vi "GEOM_VAR_HeadersArray.vi"(9 "Action":T2, 10 "GEOM_HeadersArray":T1[](array[typedef])) -> (2 "GEOM_HeadersArray out":T1[](array[typedef]))   [LabVIEW 2016]
uses:
  GEOM_VAR_action.ctl
  GEOM_ReadModeHeader.ctl
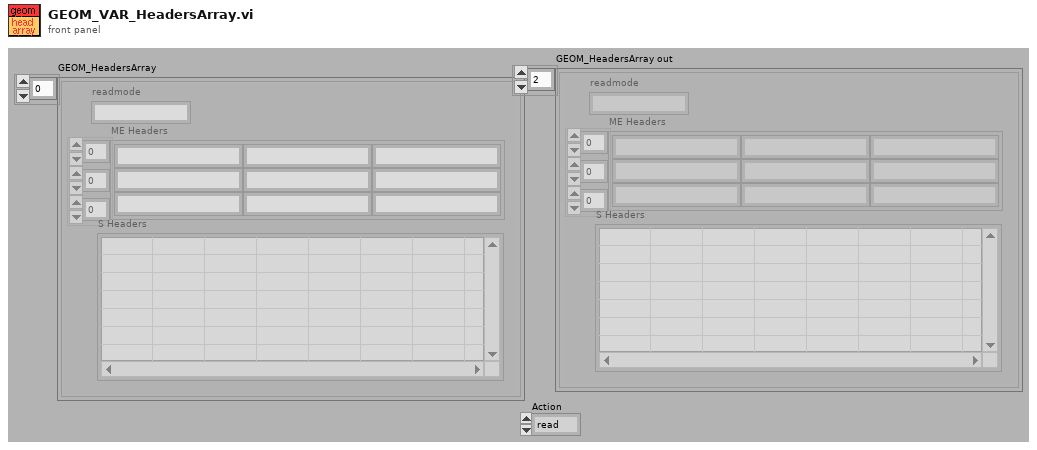
[diagram p1: front panel]
types:
  T1 = typedef "GEOM_ReadModeHeader.ctl" = cluster{"readmode":string, "ME Headers":string[][][], "S Headers":string[][]}
  T2 = typedef "GEOM_VAR_action.ctl" = enum16{"read", "write"}
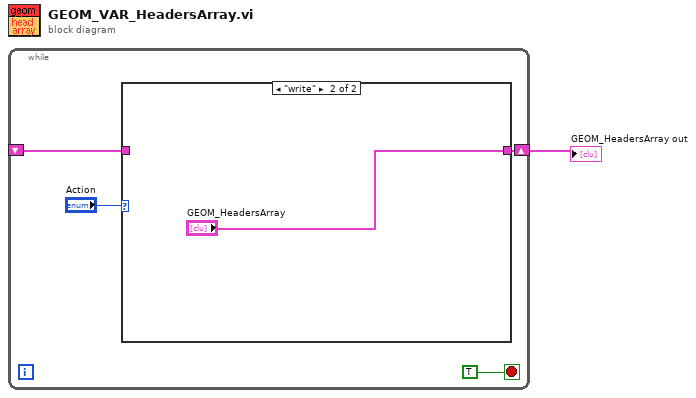
[diagram p0: block diagram]
diagram:
  n1 = while {
    shift-right: [w4] -> w1
    shift-left: _ -> [w3]
    stop <- TRUE stop-if-true
    n2 = case shown="\"write\"" "Action" {
      tunnel: [w6 "GEOM_HeadersArray"] -> w4
      tunnel: w3 -> [w6 _]
      frame "read", Default {
      }
      frame "write" {
      }
    }
  }
  "GEOM_HeadersArray out" <- w1
